vi "test.vi"() -> ()   [LabVIEW 2009]
panel:
  out "RcvQueueEmpty":bool
  out "CAN_Message out":T1 {"ID" format="%.0x"}
  in  "stop":bool
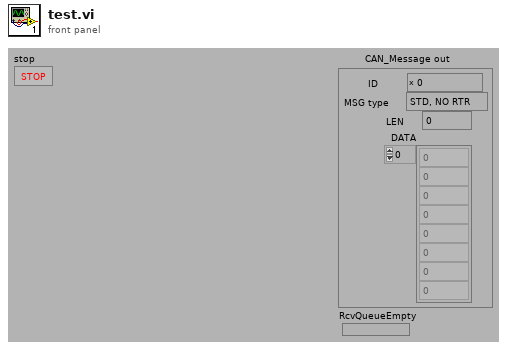
[diagram p1: front panel]
types:
  T1 = cluster{"ID":u32, "MSG type":enum8{"STD, NO RTR", "STD,RTR", "XTD, NO RTR", "XTD, RTR"}, "LEN":u8, "DATA":u8[]}
  T2 = enum16{"CAN_Baud_1M", "CAN_BAUD_500K", "CAN_BAUD_250K", "CAN_BAUD_125K", "CAN_BAUD_100K", "CAN_BAUD_50K", "CAN_BAUD_20K", "CAN_BAUD_10K", "CAN_BAUD_5K", "User"}
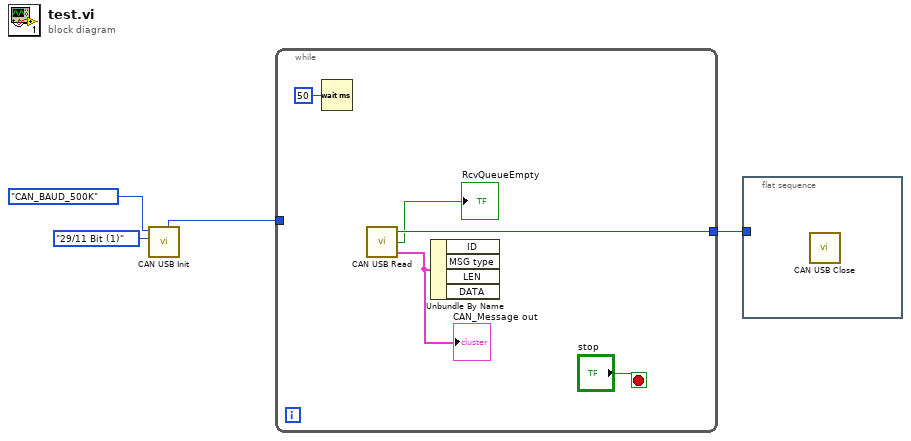
[diagram p0: block diagram]
diagram:
  n1 = call "CAN USB Init.vi"("CAN Msg Type"=enum16{"11 Bit (0)", "29/11 Bit (1)"}."29/11 Bit (1)", "BTR0BTR1"=T2."CAN_BAUD_500K") -> ("Error Number"=w2:u32)  [unwired: 7 in, 2 out]
  n2 = while {
    tunnel: w2 -> [_]
    tunnel: [w9] -> w1
    stop <- "stop" stop-if-true
    n3 = Wait (ms)(milliseconds to wait=u32 50) -> ()  [unwired: 1 out]
    n4 = call "CAN USB Read.vi"() -> ("Error Number"=w9:u32, "RcvQueueEmpty"=→"RcvQueueEmpty":bool, "CAN_Message out"=w7:T1)  [unwired: 1 in]
    "CAN_Message out" <- w7
    n5 = Unbundle By Name(w7) -> ()  [unwired: 4 out]
  }
  n6 = flat-sequence {
    tunnel: w1 -> [_]
    frame #0 {
      n7 = call "CAN USB Close.vi"() -> ()  [unwired: 1 in, 1 out]
    }
  }
